vi "Or77200_GoTo.vi"(0 "Port":refnum<visa-resource-name>, 5 "Lambda (nm)":dbl min=0.0 max=9999.9 step=0.1, 7 "Stop Ref":refnum<vi>, 9 "Move Ref":refnum<vi>, 11 "error In":errorcluster caption="error out", 12 "Lambda Ref":refnum<vi>) -> (4 "Port Out":refnum<visa-resource-name>, 6 "Lambda Out (nm)":dbl, 8 "Elapsed":u32, 15 "sortie d'erreur":errorcluster)   [LabVIEW 2019]
uses:
  <userlib>/Oriel 77200/OR77200_Goto_States.ctl
  <vilib>/Utility/config.llb/Read Key (Double).vi
  <userlib>/GenProg/WritebyWeakRefNum.vi
  <vilib>/Utility/config.llb/NI_LVConfig.lvlib
panel:
  in  "Moving":bool
  out "msBySteps":dbl
  out "Steps":i32
  in  "Stop":bool
  out "RelPos":dbl
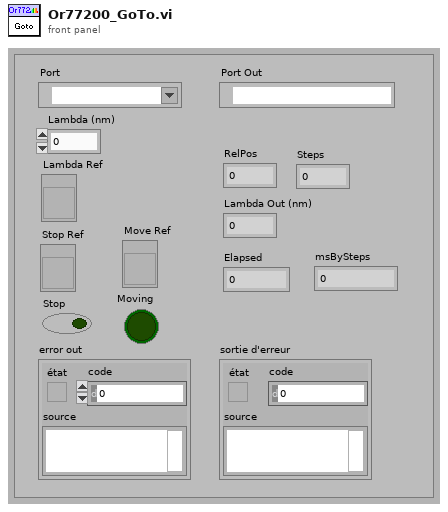
[diagram p1: front panel]
types:
  T1 = typedef "OR77200_Goto_States.ctl" = enum16{"Read Pos", "Do steps", "Check Pos", "Error"}
  T2 = typedef "NI_LVConfig.lvlib/Config Data RefNum.ctl" = refnum<k1>
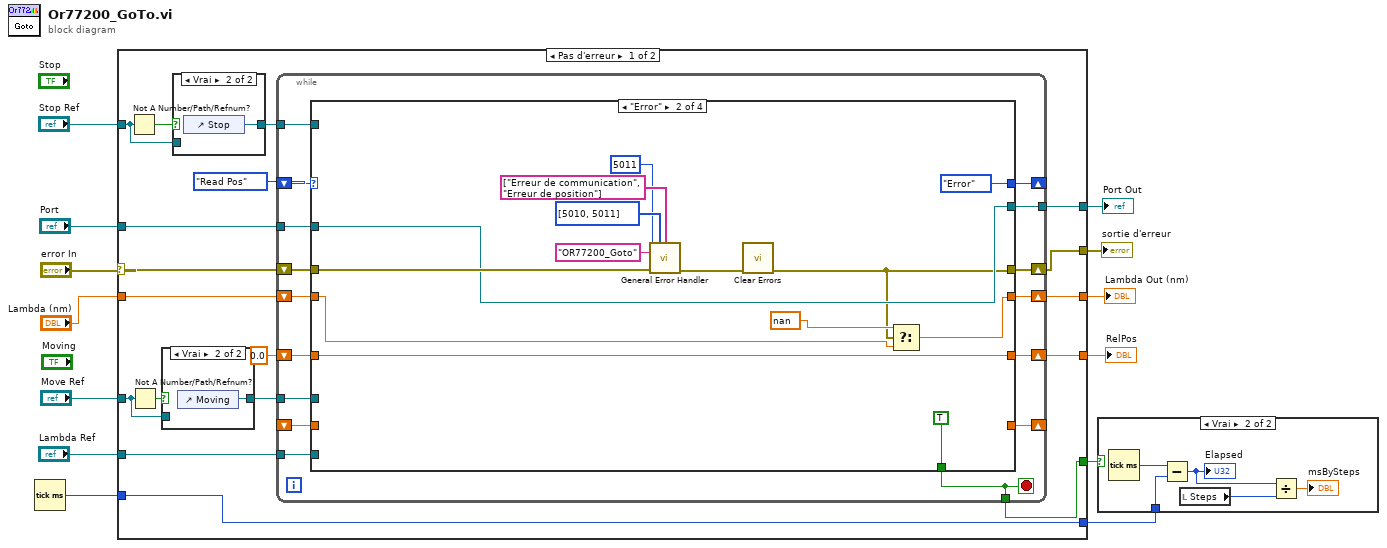
[diagram p0: block diagram]
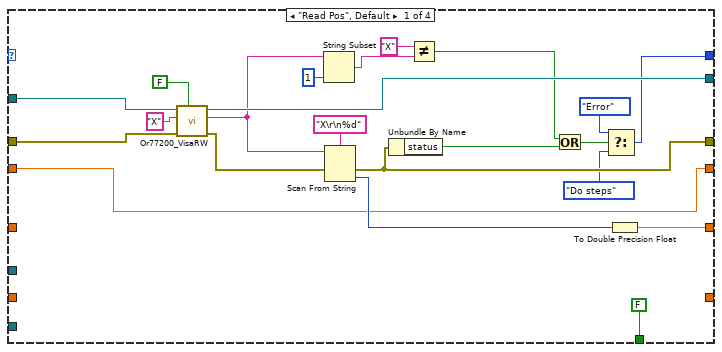
[diagram p5: hidden frame]
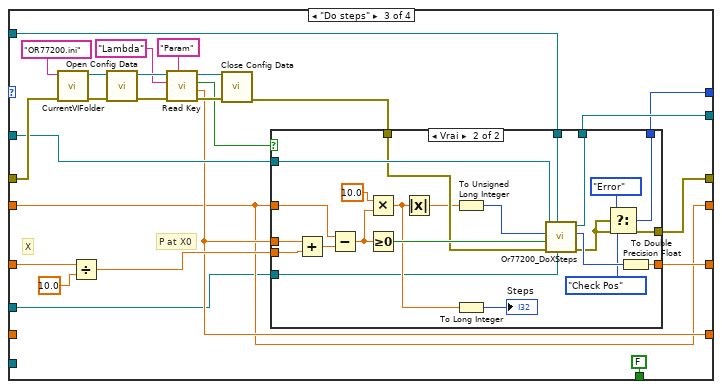
[diagram p6: hidden frame]
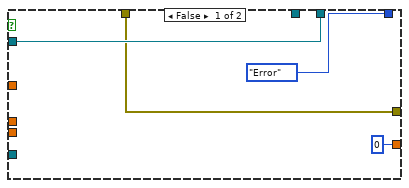
[diagram p7: hidden frame]
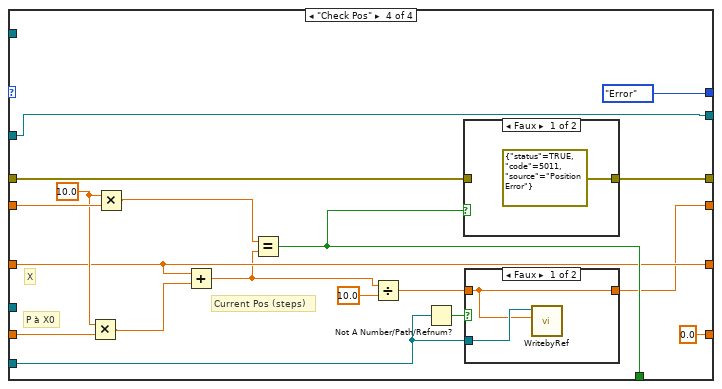
[diagram p8: hidden frame]
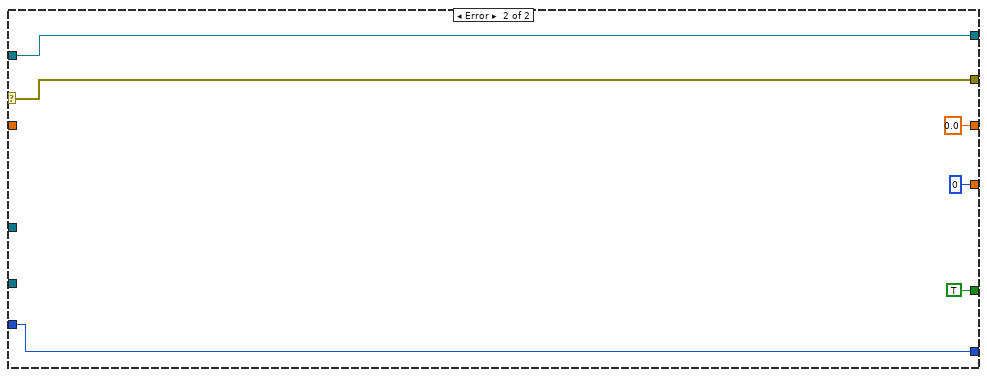
[diagram p11: hidden frame]
diagram:
  n1 = Tick Count (ms)() -> (millisecond timer value=w3:u32)
  n2 = case shown="Pas d'erreur" "error In" {
    selector: "error In" -> [w29 w166]
    tunnel: "Port" -> [w31 w167]
    tunnel: [w28 w166] -> w12
    tunnel: [w30 w167] -> w11
    tunnel: [w26 0 ("sortie 1")] -> w9
    tunnel: "Lambda (nm)" -> [w25 _]
    tunnel: "Stop Ref" -> [w21 _]
    tunnel: [w24 0.0 ("Lambda (nm)")] -> w6
    tunnel: w3 -> [w19 w162]
    tunnel: [w20 TRUE] -> w5
    tunnel: [w19 w162] -> w4
    tunnel: "Move Ref" -> [w16 _]
    tunnel: "Lambda Ref" -> [w14 _]
    frame No Error {
      n3 = Not A Number/Path/Refnum?(number/path/refnum=w21) -> (NaN/Path/Refnum?=w22:bool)
      n4 = Not A Number/Path/Refnum?(number/path/refnum=w16) -> (NaN/Path/Refnum?=w17:bool)
      n5 = case shown="Vrai" w17 {
        tunnel: [w32 w33] -> w15
        tunnel: w16 -> [w32 _]
        frame False {
        }
        frame True {
          n6 = control-ref of="Moving"() -> (w33:refnum<vi>)
        }
      }
      n7 = case shown="Vrai" w22 {
        tunnel: [w34 w35] -> w23
        tunnel: w21 -> [w34 _]
        frame False {
        }
        frame True {
          n8 = control-ref of="Stop"() -> (w35:refnum<vi>)
        }
      }
      n9 = while {
        tunnel: w31 -> [w50]
        tunnel: [w49] -> w30
        shift-right: [w46] -> _
        shift-left: OR77200_Goto_States."Read Pos" ("Énum") -> [w51]
        shift-right: [w47] -> w28
        shift-left: w29 -> [w48]
        shift-right: [w45] -> w26
        shift-left: 0.0 ("sortie 1") -> [w44]
        tunnel: w23 -> [w42]
        shift-right: [w41] -> _
        shift-left: _ -> [w40]
        shift-right: [w39] -> w24
        shift-left: w25 -> [w43]
        tunnel: [w38] -> w20
        tunnel: w15 -> [w37]
        tunnel: w14 -> [w36]
        stop <- w38 stop-if-true
        n10 = case shown="\"Error\"" w51 {
          tunnel: w50 -> [w68 w80 w99 w146]
          tunnel: [w73 w80 w98 w146] -> w49
          tunnel: w48 -> [w67 w86 w110 w150]
          tunnel: [w59 w75 w92 w152] -> w47
          tunnel: [w70 OR77200_Goto_States."Error" ("Énum") w97 OR77200_Goto_States."Error" ("Énum")] -> w46
          tunnel: [FALSE TRUE FALSE w151] -> w38
          tunnel: [w52 w78 w93 w149] -> w45
          tunnel: w44 -> [_ w78 w88 w149]
          tunnel: w43 -> [w54 w77 w90 w156]
          tunnel: w42 -> [_ _ w94 _]
          tunnel: [_ _ w91 0.0 ("value")] -> w41
          tunnel: w40 -> [_ _ _ w155]
          tunnel: [w54 w74 w90 w139] -> w39
          tunnel: w37 -> [_ _ w89 _]
          tunnel: w36 -> [_ _ _ w140]
          frame "Read Pos", Default {
            n11 = call <userlib>:"Or77200_VisaRW.vi"("Use LF-Cr"=FALSE, "error in"=w67, "Commande"="X", "Port"=w68) -> ("error out"=w65:errorcluster, "Response"=w64:string, "Port Out"=w73:refnum<visa-resource-name>)  [unwired: 4 in, 1 out]
            n12 = String Subset(string=w64, length (rest)=1 ("longueur (reste)")) -> (substring=w62:string)  [unwired: 1 in]
            n13 = Scan From String(format string="X\r\n%d" ("chaîne de format"), input string=w64, error in=w65) -> (error out=w59:errorcluster, output 1=w55:i32)  [unwired: 2 in, 2 out]
            n14 = Unbundle By Name(w59) -> ("status"=w58:bool)
            n15 = Not Equal?(x="X", y=w62) -> (x != y?=w60:bool)
            n16 = Or(x=w60, y=w58) -> (x .or. y?=w71:bool)
            n17 = Select(t=OR77200_Goto_States."Error" ("Énum"), s=w71, f=OR77200_Goto_States."Do steps" ("Énum")) -> (s? t:f=w70:T1)
            n18 = To Double Precision Float(number=w55) -> (double precision float=w52:dbl)
          }
          frame "Error" {
            n19 = call <vilib>:"General Error Handler.vi"("[error code] (0)"=5011, "[user-defined codes]"=i32[] [5010, 5011], "[user-defined descriptions]"=string[] ["Erreur de communication", "Erreur de position"], "[error source] (\" \")"="OR77200_Goto" ("[error source] (\" \")"), "error in (no error)"=w86) -> ("error out"=w81:errorcluster)  [unwired: 6 in, 4 out]
            n20 = call <vilib>:"Clear Errors.vi"("error in (no error)"=w81) -> ("error out"=w75:errorcluster)  [unwired: 5 in, 1 out]
            n21 = Select(t=nan ("Lambda (nm)"), s=w75, f=w77) -> (s? t:f=w74:dbl)
          }
          frame "Do steps" {
            # "P at X0"
            # "X"
            n22 = call <userlib>:"CurrentVIFolder.vi"("error in (no error)"=w110, "NomFichier"="OR77200.ini") -> ("error out"=w109:errorcluster, "Chemin"=w112:path)  [unwired: 7 in, 1 out]
            n23 = Divide(x=w88, y=10.0) -> (x/y=w101:dbl)
            n24 = call <vilib>:"Open Config Data.vi"("error in (no error)"=w109, "configuration file path"=w112) -> ("error out"=w108:errorcluster, "refnum"=w107:T2)  [unwired: 7 in, 1 out]
            n25 = call-poly <vilib>:"Read Key.vi"("section"="Param", "error in (no error)"=w108, "key"="Lambda", "refnum"=w107) -> ("error out"=w104:errorcluster, "value"=w91:dbl, "found?"=w96:bool, "refnum out"=w103:T2)  [unwired: 4 in]
            n26 = call <vilib>:"Close Config Data.vi"("error in (no error)"=w104, "refnum"=w103) -> ("error out"=w95:errorcluster)  [unwired: 8 in, 1 out]
            n27 = case shown="Vrai" w96 {
              tunnel: w101 -> [_ w138]
              tunnel: w90 -> [_ w137]
              tunnel: w99 -> [w116 w131]
              tunnel: [w116 w130] -> w98
              tunnel: [OR77200_Goto_States."Error" ("Énum") w124] -> w97
              tunnel: w91 -> [_ w129]
              tunnel: w95 -> [w113 w122]
              tunnel: w94 -> [_ w128]
              tunnel: [0 ("sortie 1") w117] -> w93
              tunnel: [w113 w126] -> w92
              tunnel: w89 -> [_ w118]
              frame False {
              }
              frame True {
                n28 = Add(x=w129, y=w138) -> (x+y=w136:dbl)
                n29 = Subtract(x=w137, y=w136) -> (x-y=w134:dbl)
                n30 = Multiply(x=10.0, y=w134) -> (x*y=w120:dbl)
                n31 = Greater Or Equal To 0?(x=w134) -> (x >= 0?=w135:bool)
                n32 = Absolute Value(x=w120) -> (abs(x)=w121:dbl)
                n33 = To Unsigned Long Integer(number=w121) -> (unsigned 32bit integer=w132:u32)
                n34 = To Long Integer(number=w120) -> (32bit integer=→"Steps":i32)
                n35 = call <userlib>:"Or77200_DoXSteps.vi"("MoveRef"=w118, "Stop Ref"=w128, "error In"=w122, "Dir (Dec:F)"=w135, "Steps"=w132, "Port"=w131) -> ("sortie d'erreur"=w126:errorcluster, "sortie 1"=w127:i32, "Port Out"=w130:refnum<visa-resource-name>)  [unwired: 3 in]
                n36 = Select(t=OR77200_Goto_States."Error" ("Énum"), s=w126, f=OR77200_Goto_States."Check Pos" ("Énum")) -> (s? t:f=w124:T1)
                n37 = To Double Precision Float(number=w127) -> (double precision float=w117:dbl)
              }
            }
          }
          frame "Check Pos" {
            w154 = 10.0
            # "Current Pos (steps)"
            # "X"
            # "P à X0"
            n38 = Multiply(x=w154, y=w155) -> (x*y=w144:dbl)
            n39 = Multiply(x=w154, y=w156) -> (x*y=w145:dbl)
            n40 = Add(x=w149, y=w144) -> (x+y=w143:dbl)
            n41 = Equal?(x=w145, y=w143) -> (x = y?=w151:bool)
            n42 = Divide(x=w143, y=10.0) -> (x/y=w142:dbl)
            n43 = Not A Number/Path/Refnum?(number/path/refnum=w140) -> (NaN/Path/Refnum?=w141:bool)
            n44 = case shown="Faux" w151 {
              tunnel: [errorcluster {"status"=TRUE, "code"=5011, "source"="Position Error"} ("sortie d'erreur") w161] -> w152
              tunnel: w150 -> [_ w161]
              frame False {
              }
              frame True {
              }
            }
            n45 = case shown="Faux" w141 {
              tunnel: w142 -> [w157 w159]
              tunnel: w140 -> [w158 _]
              tunnel: [w157 w159] -> w139
              frame False {
                n46 = call-poly <userlib>:"WritebyRef.vi"("Valeur"=w157, "Control Ref"=w158) -> ()  [unwired: 9 in, 1 out]
              }
              frame True {
              }
            }
          }
        }
      }
    }
    frame Error {
    }
  }
  "sortie d'erreur" <- w12
  "Port Out" <- w11
  "RelPos" <- w9
  "Lambda Out (nm)" <- w6
  n47 = case shown="Vrai" w5 {
    tunnel: w4 -> [_ w171]
    frame False {
    }
    frame True {
      n48 = Tick Count (ms)() -> (millisecond timer value=w172:u32)
      n49 = Subtract(x=w172, y=w171) -> (x-y=w170:u32)
      "Elapsed" <- w170
      n50 = local read "Steps"() -> (w169:i32)
      n51 = Divide(x=w170, y=w169) -> (x/y=→"msBySteps":dbl)
    }
  }
